vi "getCells.vi"(8 "error in (no error)":errorcluster, 11 "xwpfTable in":refnum<class "xwpfTable.lvclass">) -> (0 "error out":errorcluster, 3 "xwpfTable out":refnum<class "xwpfTable.lvclass">)   [LabVIEW 2017, in "Word_Specific.lvlib" / "xwpfTable.lvclass"]
uses:
  xwpfTable.lvclass
  xwpfTable.lvclass/xwpfTable.ctl
  C:/Users/Neo/Desktop/Dev_Tools_BR/LabVIEW_NPOI/lib/NPOI 2.1.1/NPOI.OOXML.dll
  lib/NPOI 2.1.1/NPOI.OOXML.dll
  xwpfParagraph/xwpfParagraph.lvclass
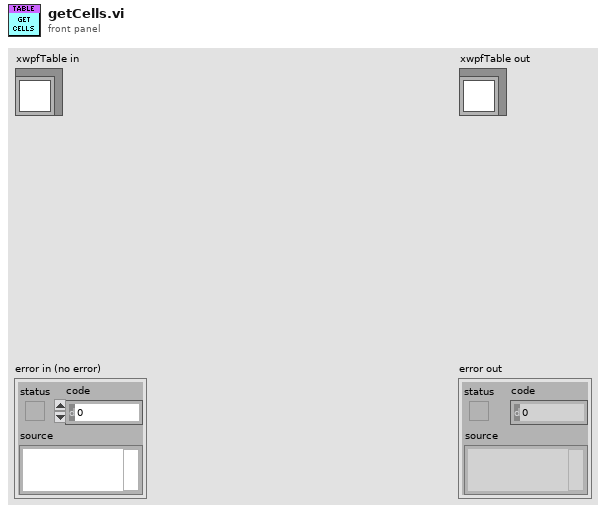
[diagram p1: front panel]
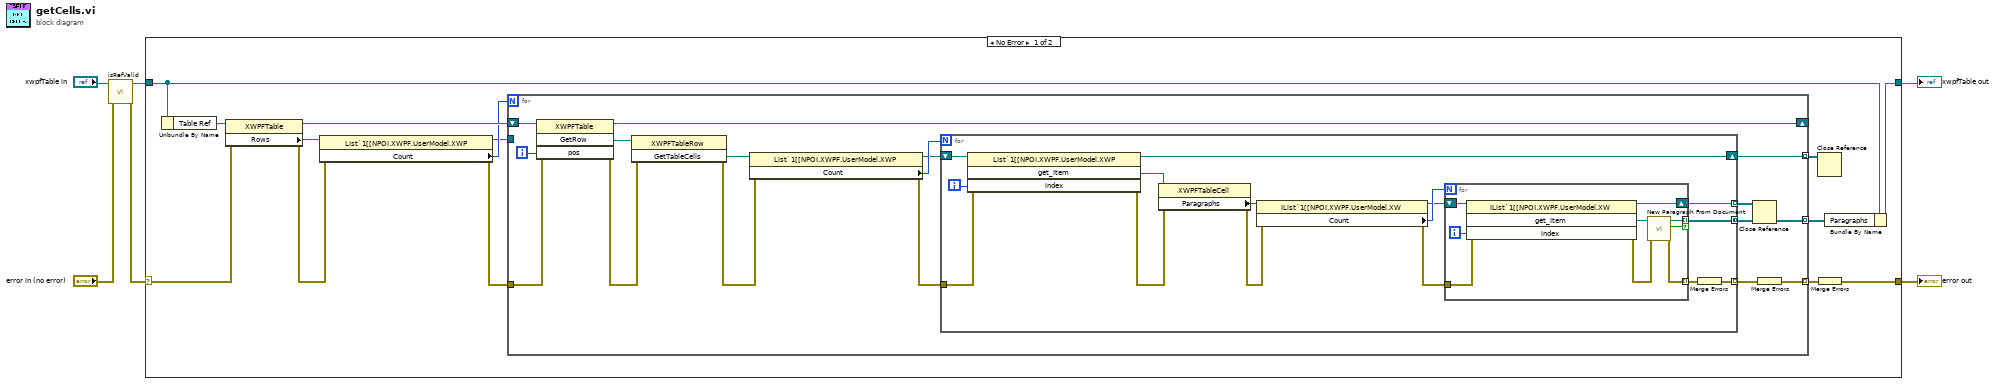
[diagram p0: block diagram]
diagram:
  n1 = call-dynamic "isRefValid.vi"("error in (no error)"="error in (no error)", "xwpfTable in"="xwpfTable in") -> ("error out"=w2:errorcluster, "xwpfTable out"=w3:refnum<class "xwpfTable.lvclass">)  [unwired: 8 in]
  n2 = case shown="No Error" w2 {
    selector: w2 -> [w13 w62]
    tunnel: [w10 w62] -> w6
    tunnel: [w9 w61] -> w4
    tunnel: w3 -> [w20 w61]
    frame No Error {
      n3 = Unbundle By Name(w20) -> ("Table Ref"=w19:refnum<k24>)
      n4 = property class="XWPFTable"(reference=w19, error in=w13) -> (reference out=w17:refnum<k24>, error out=w12:errorcluster, "Rows"=w18:refnum<k24>)
      n5 = property class="List`1[[NPOI.XWPF.UserModel.XWP"(reference=w18, error in=w12) -> (reference out=w7:refnum<k24>, error out=w14:errorcluster, "Count"=w16:i32)
      n6 = for {
        N: w16 -> [_]
        shift-right: [w35] -> _
        shift-left: w17 -> [w36]
        tunnel: [w29] -> w8 mode=indexing
        tunnel: [w28] -> w15 mode=indexing
        tunnel: [w27] -> w11 mode=indexing
        tunnel: w14 -> [w23]
        tunnel: w7 -> [_]
        i -> [w34]
        n7 = invoke class="XWPFTable" method="GetRow"(reference=w36, error in=w23, "pos"=w34) -> (reference out=w35:refnum<k24>, error out=w26:errorcluster, "GetRow"=w33:refnum<k24>)  [unwired: 1 in, 1 out]
        n8 = invoke class="XWPFTableRow" method="GetTableCells"(reference=w33, error in=w26) -> (error out=w25:errorcluster, "GetTableCells"=w32:refnum<k24>)  [unwired: 1 in, 1 out]
        n9 = property class="List`1[[NPOI.XWPF.UserModel.XWP"(reference=w32, error in=w25) -> (reference out=w22:refnum<k24>, error out=w24:errorcluster, "Count"=w31:i32)
        n10 = for {
          N: w31 -> [_]
          shift-right: [w50] -> w28
          shift-left: w22 -> [w51]
          tunnel: [w44] -> w29 mode=concatenating
          tunnel: [w43] -> w30 mode=indexing
          tunnel: [w42] -> w21 mode=indexing
          tunnel: w24 -> [w39]
          i -> [w49]
          n11 = invoke class="List`1[[NPOI.XWPF.UserModel.XWP" method="get_Item"(reference=w51, error in=w39, "index"=w49) -> (reference out=w50:refnum<k24>, error out=w41:errorcluster, "get_Item"=w48:refnum<k24>)  [unwired: 1 in, 1 out]
          n12 = property class="XWPFTableCell"(reference=w48, error in=w41) -> (error out=w40:errorcluster, "Paragraphs"=w47:refnum<k24>)  [unwired: 1 out]
          n13 = property class="IList`1[[NPOI.XWPF.UserModel.XW"(reference=w47, error in=w40) -> (reference out=w37:refnum<k24>, error out=w38:errorcluster, "Count"=w46:i32)
          n14 = for {
            N: w46 -> [_]
            shift-right: [w55] -> w42
            shift-left: w37 -> [w60]
            tunnel: [w57] -> w44 mode=indexing if=w56
            tunnel: [w52] -> w45 mode=indexing
            tunnel: w38 -> [w53]
            i -> [w59]
            n15 = invoke class="IList`1[[NPOI.XWPF.UserModel.XW" method="get_Item"(reference=w60, error in=w53, "index"=w59) -> (reference out=w55:refnum<k24>, error out=w54:errorcluster, "get_Item"=w58:refnum<k24>)  [unwired: 1 in, 1 out]
            n16 = call "New Paragraph From Document.vi"("error in (no error)"=w54, "Paragraph Ref"=w58) -> ("error out"=w52:errorcluster, "New Element Found"=w56:bool, "xwpfParagraph out"=w57:refnum<class "xwpfParagraph.lvclass">)  [unwired: 7 in]
          }
          n17 = Merge Errors(w45) -> (w43:errorcluster)
        }
        n18 = Close Reference(reference=w21) -> ()  [unwired: 1 in, 1 out]
        n19 = Merge Errors(w30) -> (w27:errorcluster)
      }
      n20 = Close Reference(reference=w15) -> ()  [unwired: 1 in, 1 out]
      n21 = Merge Errors(w11) -> (w10:errorcluster)
      n22 = Bundle By Name(cluster=w20, "Paragraphs"=w8) -> (w9:refnum<class "xwpfTable.lvclass">)
    }
    frame Error {
    }
  }
  "error out" <- w6
  "xwpfTable out" <- w4
